vi "Apply Style - input.vi"(6 "input ref":refnum<vi>, 8 "error in (no error)":errorcluster, 11 "Theme in":refnum<class "Theme.lvclass">) -> (0 "error out":errorcluster, 3 "Theme out":refnum<class "Theme.lvclass">)   [LabVIEW 2021, in "Theme.lvclass"]
doc: "Apply the theme style to an input control (double/integer digital numveric or string)\n\n<b>Code Developed By:</b> +\nDaniel Coons +\nhttps://github.com/danielcoons/tsc-pop-up"
uses:
  Theme.lvclass
  Theme.lvclass/Theme.ctl
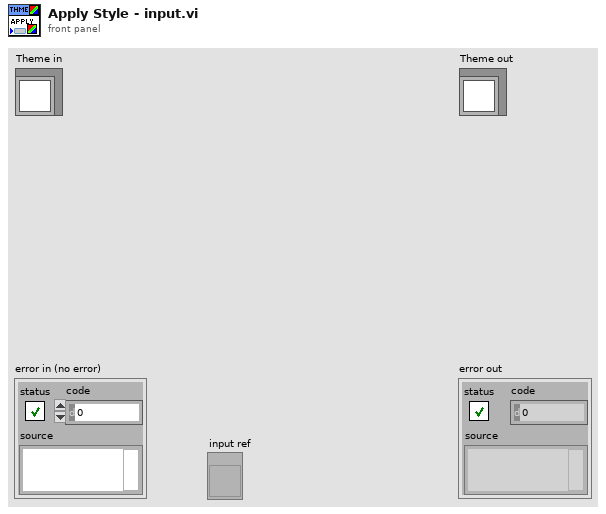
[diagram p1: front panel]
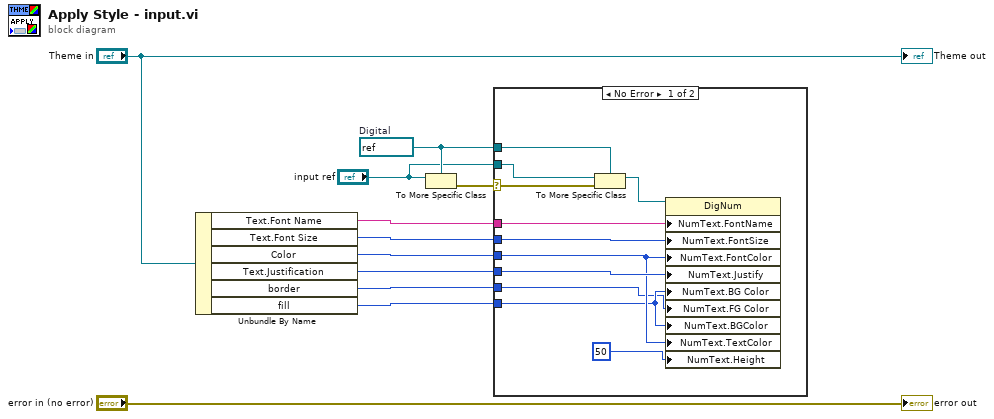
[diagram p0: block diagram]
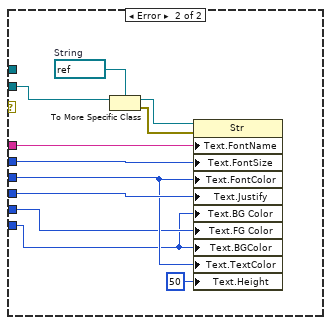
[diagram p2: hidden frame]
diagram:
  w2 = refnum<vi> refnum  # Digital
  n1 = Unbundle By Name("Theme in") -> ("Text.Font Name"=w9:string, "Text.Font Size"=w8:u32, "Color"=w7:u32, "Text.Justification"=w6:enum16{"Left", "Center", "Right"}, "border"=w5:u32, "fill"=w4:u32)
  n2 = To More Specific Class(target class=w2, reference="input ref") -> (error out=w3:errorcluster)  [unwired: 1 in, 1 out]
  n3 = case shown="No Error" w3 {
    selector: w3 -> [w19 _]
    tunnel: w9 -> [w22 w33]
    tunnel: w8 -> [w21 w32]
    tunnel: w7 -> [w15 w27]
    tunnel: w6 -> [w20 w31]
    tunnel: w5 -> [w13 w25]
    tunnel: w4 -> [w14 w24]
    tunnel: w2 -> [w18 _]
    tunnel: "input ref" -> [w17 w30]
    frame No Error {
      n4 = To More Specific Class(target class=w18, reference=w17, error in=w19) -> (specific class reference=w16:refnum<vi>)  [unwired: 1 out]
      n5 = property on="Property Node" class="DigNum"(reference=w16, "NumText.FontName"=w22, "NumText.FontSize"=w21, "NumText.FontColor"=w15, "NumText.Justify"=w20, "NumText.BG Color"=w14, "NumText.FG Color"=w13, "NumText.BGColor"=w14, "NumText.TextColor"=w15, "NumText.Height"=u32 50 ("Numeric Text.Size:Height")) -> ()  [unwired: 1 in, 2 out]
    }
    frame Error {
      w28 = refnum<vi> refnum  # String
      n6 = To More Specific Class(target class=w28, reference=w30) -> (specific class reference=w29:refnum<vi>, error out=w26:errorcluster)  [unwired: 1 in]
      n7 = property on="Property Node" class="Str"(reference=w29, error in=w26, "Text.FontName"=w33, "Text.FontSize"=w32, "Text.FontColor"=w27, "Text.Justify"=w31, "Text.BG Color"=w24, "Text.FG Color"=w25, "Text.BGColor"=w24, "Text.TextColor"=w27, "Text.Height"=u32 50 ("Text.Size:Height")) -> ()  [unwired: 2 out]
    }
  }
  "error out" <- "error in (no error)"
  "Theme out" <- "Theme in"
